vi "Get Error.vi"() -> ()   [LabVIEW 2015]
panel:
  in  "error":errorcluster
  out "error":errorcluster
  out "Error Byte":u8
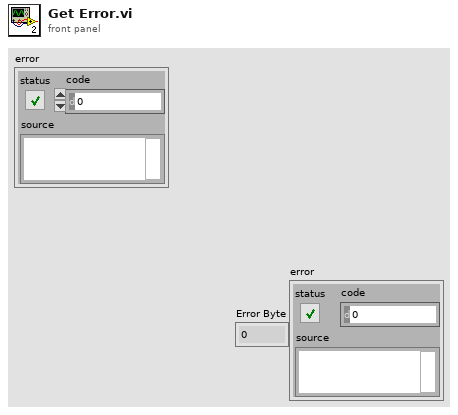
[diagram p1: front panel]
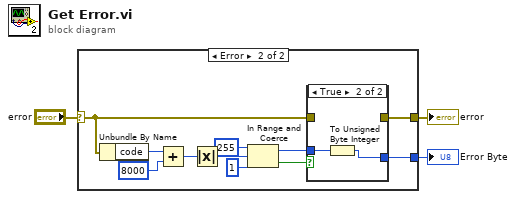
[diagram p0: block diagram]
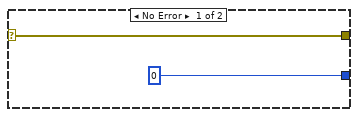
[diagram p2: hidden frame]
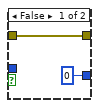
[diagram p3: hidden frame]
diagram:
  n1 = case shown="Error" "error" {
    selector: "error" -> [w4 w7]
    tunnel: [u8 0 w9] -> w3
    tunnel: [w4 w6] -> w2
    frame No Error {
    }
    frame Error {
      n2 = Unbundle By Name(w7) -> ("code"=w16:i32)
      n3 = Add(x=w16, y=8000) -> (x+y=w14:i32)
      n4 = Absolute Value(x=w14) -> (abs(x)=w13:i32)
      n5 = In Range and Coerce(upper limit=255, x=w13, lower limit=1) -> (coerced(x)=w8:i32, In Range?=w10:bool)
      n6 = case shown="True" w10 {
        tunnel: [u8 0 ("upper limit") w19] -> w9
        tunnel: w8 -> [_ w20]
        tunnel: w7 -> [w18 _]
        tunnel: [w18 _] -> w6
        frame False {
        }
        frame True {
          n7 = To Unsigned Byte Integer(number=w20) -> (unsigned 8bit integer=w19:u8)
        }
      }
    }
  }
  "Error Byte" <- w3
  "error" <- w2
